vi "cs_duplicateRows.vi"(10 "Repetitions":i32=1 min=1 step=1, 11 "Input":dbl[][](array[numeric])) -> (3 "Output":dbl[][](array[numeric]))   [LabVIEW 2013]
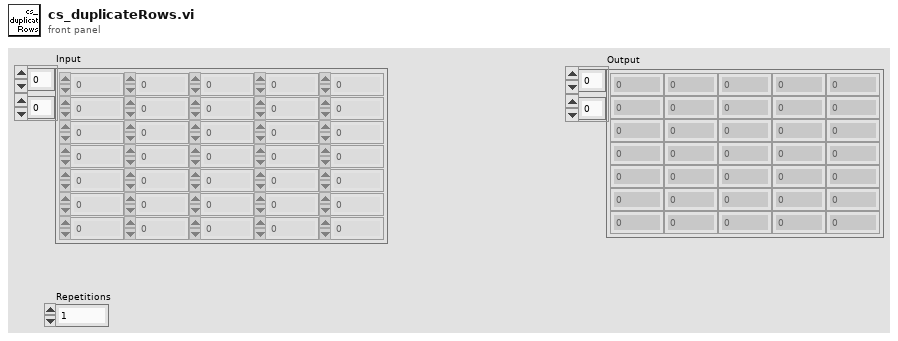
[diagram p1: front panel]
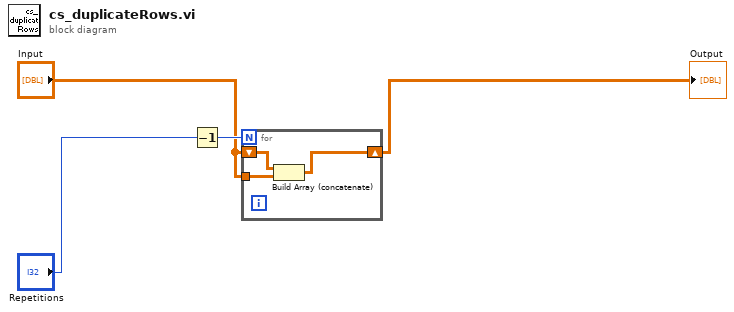
[diagram p0: block diagram]
diagram:
  n1 = Decrement(x="Repetitions") -> (x-1=w4:i32)
  n2 = for {
    N: w4 -> [_]
    shift-right: [w6] -> w2
    shift-left: "Input" -> [w7]
    tunnel: "Input" -> [w5]
    n3 = Build Array (concatenate)(w7, w5) -> (w6:dbl[][])
  }
  "Output" <- w2
